vi "[FPGA] DeltaSig Main V6_5Mod.vi"() -> ()   [LabVIEW 2015]
doc: "This VI provides a template for customizing a waveform acquisition using delta-sigma based NI C Series analog input smodules."
uses:
  <vilib>/LabVIEW Targets/FPGA/cRIO/shared/nicrio_ModuleControls/nicrio_cRIO-9234_ConfigModeRing.ctl
  <vilib>/rvi/Emulation/niFpgaGetClockAttributes.vi
  <vilib>/rvi/Emulation/niFpgaSctlEmulationGetInTimedLoop.vi
  <vilib>/rvi/Emulation/niFpgaEmulationReportErrorSimple.vi
  <vilib>/LabVIEW Targets/FPGA/cRIO/shared/nicrio_DsaDataRateApi/_nicrio_9234GetDataRate131.vi
  <vilib>/rvi/Emulation/niFpgaProcessEmulError.vi
  <vilib>/rvi/eio/common/nirviEmuTemplatePropertySet_errors.vi
  <vilib>/rvi/eio/common/nirviEmuTemplateMethod_errors.vi
  <vilib>/rvi/interface/RandomDataEmulation/niFpgaRandomDataHandleErrors.vi
  <vilib>/rvi/Emulation/niFpgaCriticalErrorInLSC.vi
  <vilib>/eio/EIOPropertyNode/EIOPropertyNode.xnode
  <vilib>/LabVIEW Targets/FPGA/cRIO/shared/nicrio_ModuleControls/nicrio_cRIO-9234_DataRatesRing2.ctl
  <vilib>/eio/EIONode/EIONode.xnode
  <vilib>/rvi/DataTransferAndStorage/Container/XNode/niFpgaContainer.xnode
  <vilib>/rvi/interface/RandomDataEmulation/nirviRandomDataFpgaReadWriteTemplate.vi
  <vilib>/rvi/eio/common/nirviEmuTemplatePropertyGet_errors.vi
  <vilib>/rvi/eio/common/nirviEmuTemplatePropertyGet_noerrors.vi
  <vilib>/rvi/eio/common/nirviEmuTemplatePropertySet_noerrors.vi
panel:
  in  "Array Input Config":T1[](array[typedef])=[0, 0, 0, 0, 0, 0, 0, 0, 0, 0, 0, 0, 0, 0, 0, 0, 0, 0, 0, 0, 0, 0, 0, 0] items=["AC Coupled", "DC Coupled", "IEPE AC Coupled"]
  out "oclk freq":u32
  out "oclk div":u32
  out "oclk mult":u32
  in  "data rate (S/s)":u32
  in  "Chan Scale Array":sgl[](array[numeric])=[0.0, 0.0, 0.0, 0.0, 0.0, 0.0, 0.0, 0.0, 0.0, 0.0, 0.0, 0.0, 0.0, 0.0, 0.0, 0.0, 0.0, 0.0, 0.0, 0.0, 0.0, 0.0, 0.0, 0.0, 0.0, 0.0, 0.0, 0.0, 0.0, 0.0, 0.0, 0.0, 0.0, 0.0, 0.0, 0.0, 0.0, 0.0, 0.0, 0.0]
  out "Chan Count":bool
  out "Acq Loop Ticks":u32
  out "FPGA Error":errorcluster
  out "Module Underflow":bool
  out "Finished":bool
  in  "Number of Channels":i32=24
  in  "Samps per Chan [Finite]":i32=5120
  out "First Read":bool
  in  "Acquisition Type":enum16{"Finite Samples", "Continuous Samples"}(ring)
  out "DMA FIFO Full":bool
  in  "stop":bool
  # "Array size fixed at 40\nelements but may be \nexpanded if needed"
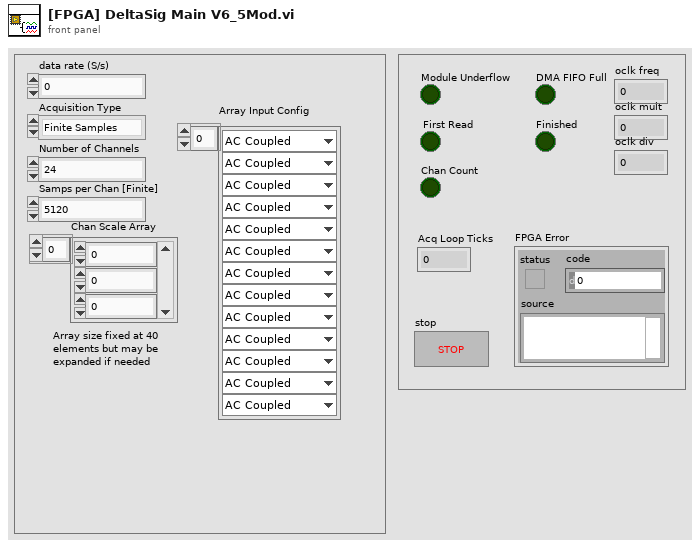
[diagram p1: front panel]
types:
  T1 = typedef "nicrio_cRIO-9234_ConfigModeRing.ctl" = u8
  T2 = typedef "nicrio_cRIO-9234_DataRatesRing2.ctl" = u8
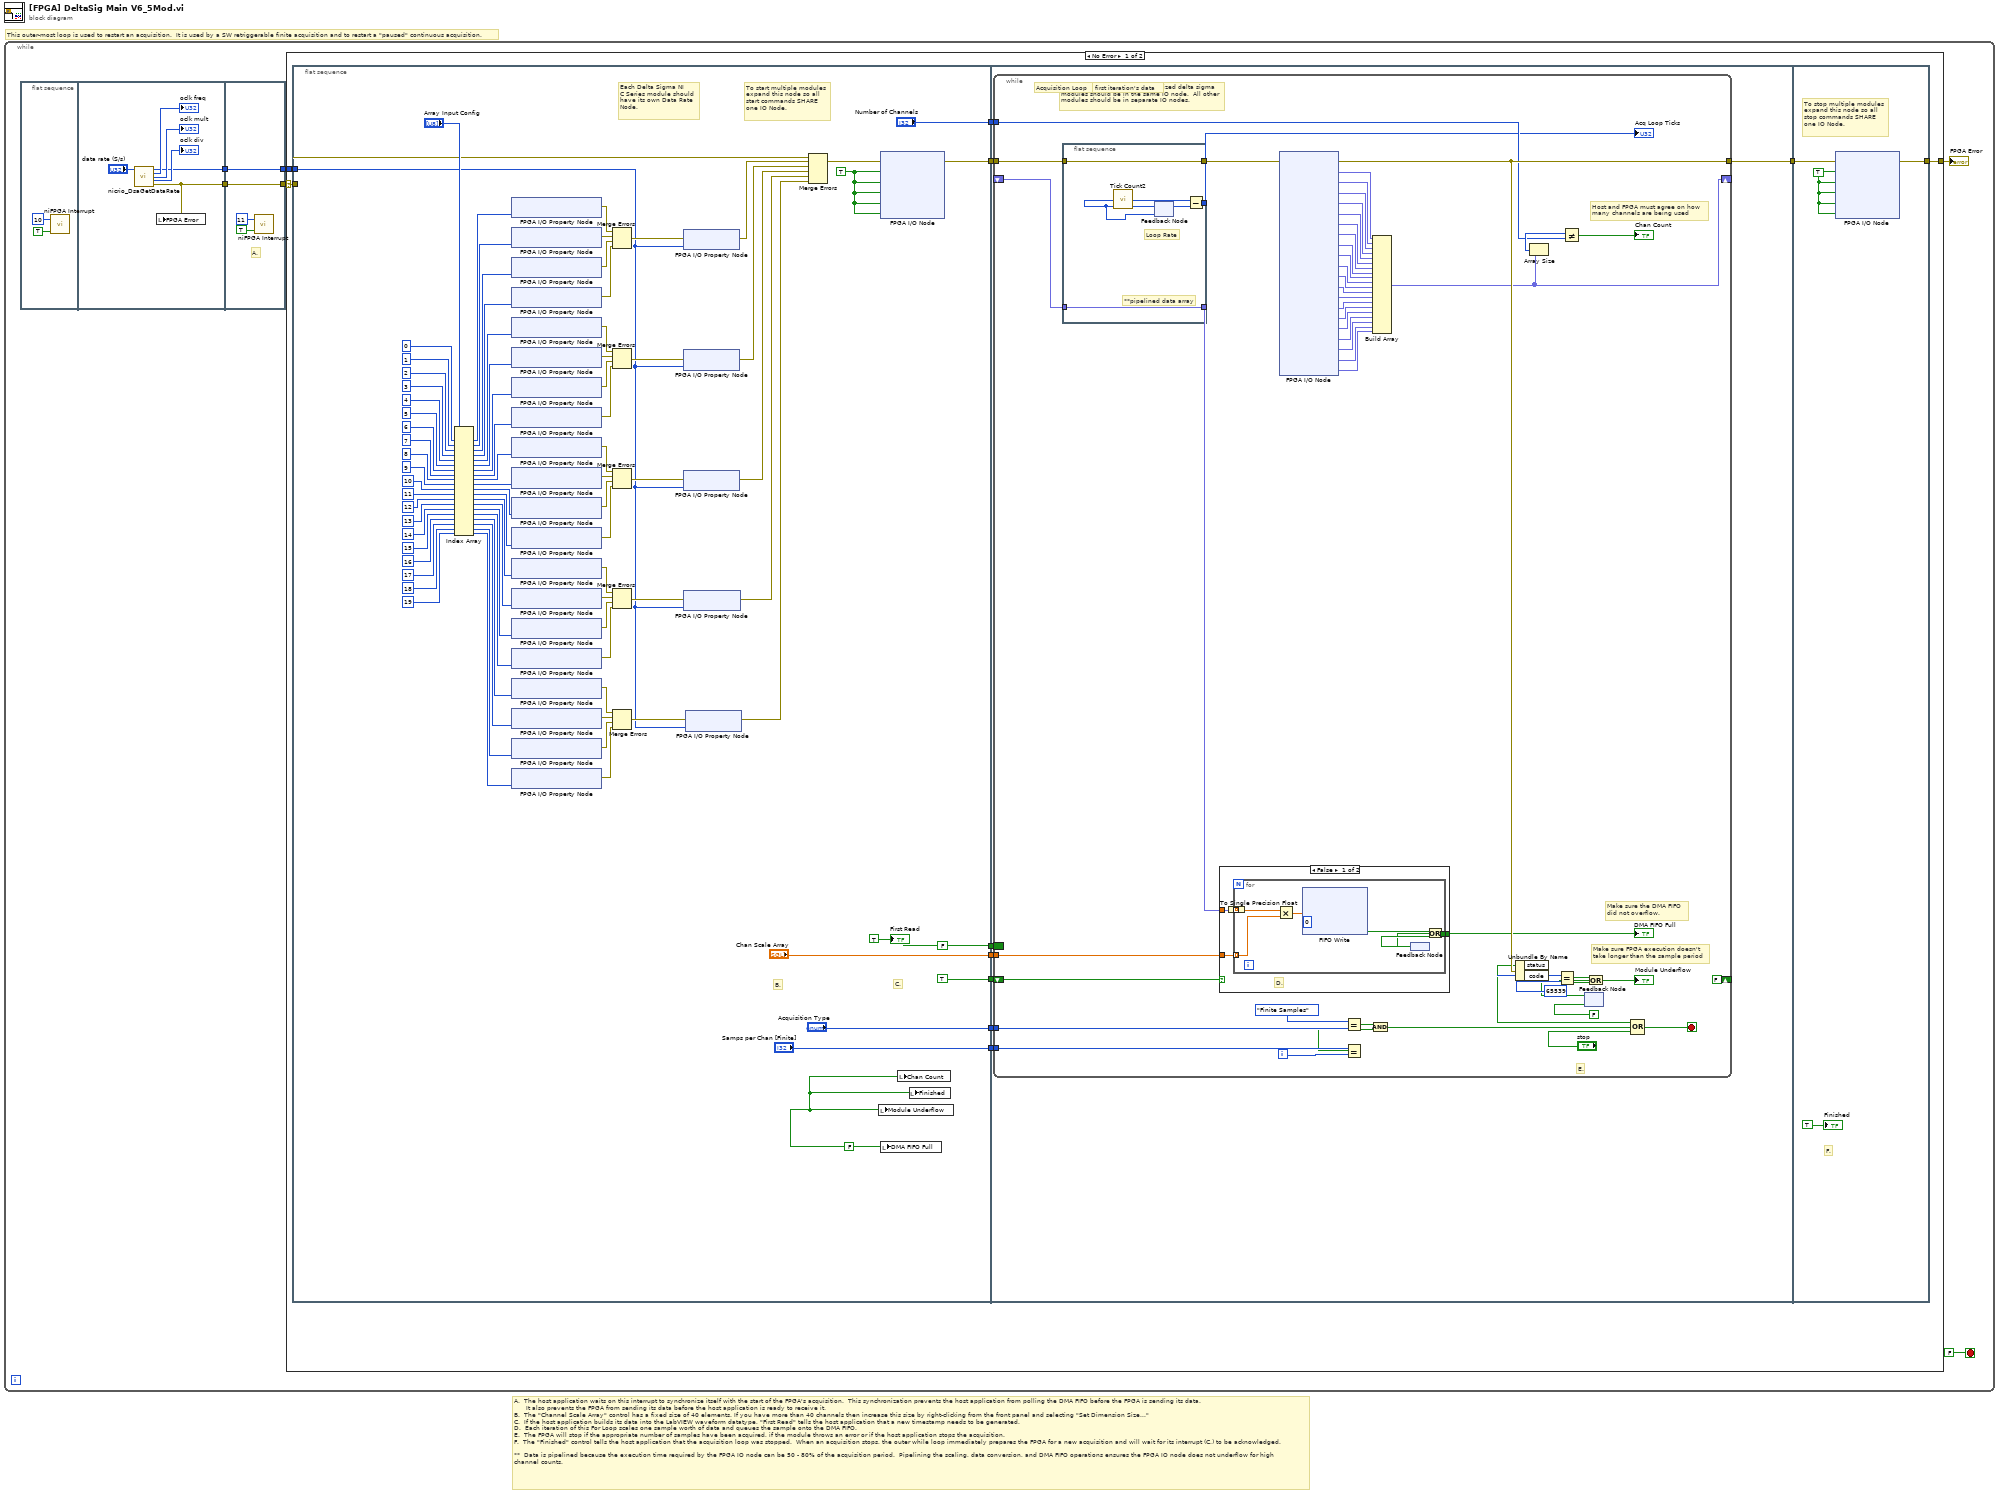
[diagram p0: block diagram]
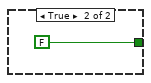
[diagram p2: hidden frame]
diagram:
  # "A.  The host application waits on this interrupt to synchronize itself with the start of the FPGA's acquisition.  This synchronization prevents the host application from polling the DMA FIFO before the FPGA is sending its data.\n      It also prevents the FPGA from sending its data before the host application is ready to receive it.\nB.  The \"Channel Scale Array\" control has a fixed size of 40 elements. If you have more than 40 channels then increase this size by right-clicking from the front panel and selecting \"Set Dimension Size...\"\nC.  If the host application builds its data into the LabVIEW waveform datatype, \"First Read\" tells the host application that a new timestamp needs to be generated.\nD.  Each iteration of this For Loop scales one sample worth of data and queues the sample onto the DMA FIFO.  \nE.  The FPGA will stop if the appropriate number of samples have been acquired, if the module throws an error or if the host application stops the acquisition.  \nF.  The \"Finished\" control tells the host application that the acquisition loop was stopped.  When an acquisition stops, the outer while loop immediately prepares the FPGA for a new acquisition and will wait for its interrupt (C.) to be acknowledged.\n\n**  Data is pipelined because the execution time required by the FPGA IO node can be 50 - 80% of the acquisition period.  Pipelining the scaling, data conversion, and DMA FIFO operations ensures the FPGA IO node does not underflow for high\nchannel counts."
  # "This outer-most loop is used to restart an acquisition.  It is used by a SW retriggerable finite acquisition and to restart a \"paused\" continuous acquisition."
  n1 = while {
    stop <- FALSE stop-if-true
    n2 = flat-sequence {
      tunnel: [w10] -> w2
      tunnel: [w11] -> w1
      tunnel: [w18] -> w3
      tunnel: [w15] -> w4
      tunnel: w2 -> [w15]
      tunnel: w1 -> [w18]
      frame #0 {
        n3 = call <vilib>:"niFPGA Interrupt.vi"("Wait Until Cleared (F)"=TRUE ("Wait Until Cleared"), "IRQ Number (0)"=u8 10 ("IRQ Number")) -> ()  [unwired: 1 in]
      }
      frame #1 {
        n4 = call-poly <vilib>:"nicrio_DsaGetDataRate.vi"("data rate (S/s)"="data rate (S/s)") -> ("data rate"=w11:T2, "oclk freq"=→"oclk freq":u32, "oclk mult"=→"oclk mult":u32, "oclk div"=→"oclk div":u32, "error out"=w10:errorcluster)  [unwired: 10 in]
        n5 = local write "FPGA Error"(w10) -> ()
      }
      frame #2 {
        # "A."
        n6 = call <vilib>:"niFPGA Interrupt.vi"("Wait Until Cleared (F)"=TRUE ("Wait Until Cleared"), "IRQ Number (0)"=u8 11 ("IRQ Number")) -> ()  [unwired: 1 in]
      }
    }
    n7 = case shown="No Error" w4 {
      selector: w4 -> [w19 w193]
      tunnel: [w21 w193] -> w5
      tunnel: w3 -> [w20 _]
      frame No Error {
        n8 = flat-sequence {
          tunnel: [w113] -> w29
          tunnel: ["Chan Scale Array"] -> w28
          tunnel: ["Acquisition Type"] -> w27
          tunnel: ["Samps per Chan [Finite]"] -> w26
          tunnel: ["Number of Channels"] -> w25
          tunnel: [TRUE ("t")] -> w24
          tunnel: [FALSE] -> w23
          tunnel: w20 -> [w33]
          tunnel: w19 -> [w85]
          tunnel: w29 -> [w120]
          tunnel: w28 -> [w119]
          tunnel: w27 -> [w117]
          tunnel: w26 -> [w116]
          tunnel: w25 -> [w121]
          tunnel: w24 -> [w118]
          tunnel: [w115] -> w22
          tunnel: w23 -> [w114]
          tunnel: w22 -> [w191]
          tunnel: [w190] -> w21
          frame #0 {
            w111 = FALSE ("Module Underflow")
            w73 = TRUE ("Mod1/Start")
            # "To start multiple modules\nexpand this node so all\nstart commands SHARE\none IO Node."
            # "C."
            # "B."
            # "Each Delta Sigma NI \nC Series module should \nhave its own Data Rate \nNode."
            n9 = Index Array(array="Array Input Config", index #1=0 ("index"), index #2=1 ("index"), index #3=2 ("index"), index #4=3 ("index"), index #5=4 ("index"), index #6=5 ("index"), index #7=6 ("index"), index #8=7 ("index"), index #9=8 ("index"), index #10=9 ("index"), index #11=10 ("index"), index #12=11 ("index"), index #13=12 ("index"), index #14=13 ("index"), index #15=14 ("index"), index #16=15 ("index"), index #17=16 ("index"), index #18=17 ("index"), index #19=18 ("index"), index #20=19 ("index")) -> (element #1=w103:T1, element #2=w102:T1, element #3=w101:T1, element #4=w100:T1, element #5=w81:T1, element #6=w80:T1, element #7=w79:T1, element #8=w78:T1, element #9=w60:T1, element #10=w59:T1, element #11=w58:T1, element #12=w57:T1, element #13=w56:T1, element #14=w54:T1, element #15=w53:T1, element #16=w52:T1, element #17=w51:T1, element #18=w50:T1, element #19=w49:T1, element #20=w48:T1)
            n10 = xnode "FPGA I/O Property Node"("Input Configuration"=w103) -> ("error out"=w96:errorcluster)  [unwired: 2 in, 1 out]
            n11 = xnode "FPGA I/O Property Node"("Input Configuration"=w102) -> ("error out"=w95:errorcluster)  [unwired: 2 in, 1 out]
            n12 = xnode "FPGA I/O Property Node"("Input Configuration"=w101) -> ("error out"=w94:errorcluster)  [unwired: 2 in, 1 out]
            n13 = xnode "FPGA I/O Property Node"("Input Configuration"=w100) -> ("error out"=w93:errorcluster)  [unwired: 2 in, 1 out]
            n14 = xnode "FPGA I/O Property Node"("Input Configuration"=w81) -> ("error out"=w90:errorcluster)  [unwired: 2 in, 1 out]
            n15 = xnode "FPGA I/O Property Node"("Input Configuration"=w80) -> ("error out"=w89:errorcluster)  [unwired: 2 in, 1 out]
            n16 = xnode "FPGA I/O Property Node"("Input Configuration"=w79) -> ("error out"=w88:errorcluster)  [unwired: 2 in, 1 out]
            n17 = xnode "FPGA I/O Property Node"("Input Configuration"=w78) -> ("error out"=w87:errorcluster)  [unwired: 2 in, 1 out]
            n18 = xnode "FPGA I/O Property Node"("Input Configuration"=w60) -> ("error out"=w72:errorcluster)  [unwired: 2 in, 1 out]
            n19 = xnode "FPGA I/O Property Node"("Input Configuration"=w59) -> ("error out"=w71:errorcluster)  [unwired: 2 in, 1 out]
            n20 = xnode "FPGA I/O Property Node"("Input Configuration"=w58) -> ("error out"=w70:errorcluster)  [unwired: 2 in, 1 out]
            n21 = xnode "FPGA I/O Property Node"("Input Configuration"=w57) -> ("error out"=w69:errorcluster)  [unwired: 2 in, 1 out]
            n22 = xnode "FPGA I/O Property Node"("Input Configuration"=w56) -> ("error out"=w68:errorcluster)  [unwired: 2 in, 1 out]
            n23 = xnode "FPGA I/O Property Node"("Input Configuration"=w54) -> ("error out"=w67:errorcluster)  [unwired: 2 in, 1 out]
            n24 = xnode "FPGA I/O Property Node"("Input Configuration"=w53) -> ("error out"=w66:errorcluster)  [unwired: 2 in, 1 out]
            n25 = xnode "FPGA I/O Property Node"("Input Configuration"=w52) -> ("error out"=w65:errorcluster)  [unwired: 2 in, 1 out]
            n26 = xnode "FPGA I/O Property Node"("Input Configuration"=w51) -> ("error out"=w64:errorcluster)  [unwired: 2 in, 1 out]
            n27 = xnode "FPGA I/O Property Node"("Input Configuration"=w50) -> ("error out"=w63:errorcluster)  [unwired: 2 in, 1 out]
            n28 = xnode "FPGA I/O Property Node"("Input Configuration"=w49) -> ("error out"=w62:errorcluster)  [unwired: 2 in, 1 out]
            n29 = xnode "FPGA I/O Property Node"("Input Configuration"=w48) -> ("error out"=w61:errorcluster)  [unwired: 2 in, 1 out]
            n30 = Merge Errors(w96, w95, w94, w93) -> (w92:errorcluster)
            n31 = Merge Errors(w90, w89, w88, w87) -> (w86:errorcluster)
            n32 = Merge Errors(w72, w71, w70, w69) -> (w55:errorcluster)
            n33 = Merge Errors(w68, w67, w66, w65) -> (w35:errorcluster)
            n34 = Merge Errors(w64, w63, w62, w61) -> (w34:errorcluster)
            n35 = xnode "FPGA I/O Property Node"("error in"=w92, "Data Rate"=w33) -> ("error out"=w83:errorcluster)  [unwired: 1 in, 1 out]
            n36 = xnode "FPGA I/O Property Node"("error in"=w86, "Data Rate"=w33) -> ("error out"=w82:errorcluster)  [unwired: 1 in, 1 out]
            n37 = xnode "FPGA I/O Property Node"("error in"=w55, "Data Rate"=w33) -> ("error out"=w32:errorcluster)  [unwired: 1 in, 1 out]
            n38 = xnode "FPGA I/O Property Node"("error in"=w35, "Data Rate"=w33) -> ("error out"=w31:errorcluster)  [unwired: 1 in, 1 out]
            n39 = xnode "FPGA I/O Property Node"("error in"=w34, "Data Rate"=w33) -> ("error out"=w30:errorcluster)  [unwired: 1 in, 1 out]
            n40 = Merge Errors(w85, w83, w82, w32, w31, w30) -> (w84:errorcluster)
            n41 = local write "Module Underflow"(w111) -> ()
            n42 = xnode "FPGA I/O Node"("error in"=w84, "Mod1/Start"=w73, "Mod2/Start"=w73, "Mod3/Start"=w73, "Mod4/Start"=w73, "Mod5/Start"=w73) -> ("error out"=w113:errorcluster)  [unwired: 5 in, 5 out]
            n43 = local write "DMA FIFO Full"(w111) -> ()
            n44 = local write "Chan Count"(w111) -> ()
            n45 = local write "Finished"(w111) -> ()
            "First Read" <- TRUE ("First Read")
          }
          frame #1 {
            n46 = while {
              tunnel: w120 -> [w161]
              tunnel: [w166] -> w115
              tunnel: w117 -> [w168]
              tunnel: w116 -> [w167]
              shift-right: [w141] -> _
              shift-left: _ -> [w154]
              tunnel: w121 -> [w163]
              tunnel: w119 -> [w155]
              shift-right: [FALSE ("t")] -> _
              shift-left: w118 -> [w153]
              border: w114 -> [_]
              i -> [w151]
              stop <- w138 stop-if-true
              # "Add channels here.  All synchronized delta sigma\nmodules should be in the same IO node.  All other\nmodules should be in separate IO nodes."
              # "Do not DMA first iteration's data"
              # "Acquisition Loop"
              # "E."
              # "Host and FPGA must agree on how \nmany channels are being used"
              # "Make sure the DMA FIFO\ndid not overflow."
              # "Make sure FPGA execution doesn't\ntake longer than the sample period"
              n47 = flat-sequence {
                tunnel: [w188] -> w160
                tunnel: w161 -> [w188]
                tunnel: [w185] -> w159
                tunnel: w154 -> [w184]
                tunnel: [w184] -> w140
                frame #0 {
                  # "**pipelined data array"
                  # "Loop Rate"
                  n48 = call "Tick Count2"() -> ("Tick Count(Ticks)"=w187:u32)
                  n49 = feedback-in #1(w187) -> ()
                  n50 = feedback #1(w187) -> (w186:u32)
                  n51 = Subtract(x=w187, y=w186) -> (x-y=w185:u32)
                }
              }
              n52 = To Single Precision Float(number=w140) -> (single precision float=w139:sgl[])
              n53 = case shown="False" w153 {
                tunnel: [w175 FALSE] -> w165
                tunnel: w155 -> [w174 _]
                tunnel: w139 -> [w173 _]
                frame False {
                  # "D."
                  n54 = for {
                    tunnel: [w180] -> w175
                    tunnel: w173 -> [w178] mode=indexing
                    tunnel: w174 -> [w177] mode=indexing
                    n55 = Multiply(x=w178, y=w177) -> (x*y=w176:sgl)
                    n56 = xnode ("FIFO Write")("Element"=w176, "Timeout"=0) -> ("Timed Out?"=w182:bool)  [unwired: 1 in, 1 out]
                    n57 = feedback #2() -> (w181:bool)
                    n58 = Or(x=w182, y=w181) -> (x .or. y?=w180:bool)
                    n59 = feedback-in #2(w180) -> ()
                  }
                }
                frame True {
                }
              }
              "DMA FIFO Full" <- w165
              n60 = xnode "FPGA I/O Node"("error in"=w160) -> ("error out"=w166:errorcluster, "Mod1/AI0"=w158:fxp<+/-,24,4>, "Mod1/AI1"=w150:fxp<+/-,24,4>, "Mod1/AI2"=w157:fxp<+/-,24,4>, "Mod1/AI3"=w156:fxp<+/-,24,4>, "Mod2/AI0"=w137:fxp<+/-,24,4>, "Mod2/AI1"=w136:fxp<+/-,24,4>, "Mod2/AI2"=w135:fxp<+/-,24,4>, "Mod2/AI3"=w134:fxp<+/-,24,4>, "Mod3/AI0"=w133:fxp<+/-,24,4>, "Mod3/AI1"=w132:fxp<+/-,24,4>, "Mod3/AI2"=w131:fxp<+/-,24,4>, "Mod3/AI3"=w130:fxp<+/-,24,4>, "Mod4/AI0"=w129:fxp<+/-,24,4>, "Mod4/AI1"=w128:fxp<+/-,24,4>, "Mod4/AI2"=w127:fxp<+/-,24,4>, "Mod4/AI3"=w126:fxp<+/-,24,4>, "Mod5/AI0"=w125:fxp<+/-,24,4>, "Mod5/AI1"=w124:fxp<+/-,24,4>, "Mod5/AI2"=w123:fxp<+/-,24,4>, "Mod5/AI3"=w122:fxp<+/-,24,4>)  [unwired: 20 in, 20 out]
              n61 = Equal?(x=enum16{"Finite Samples", "Continuous Samples"}."Finite Samples" ("y"), y=w168) -> (x = y?=w144:bool)
              n62 = Equal?(x=w167, y=w151) -> (x = y?=w143:bool)
              n63 = And(x=w144, y=w143) -> (x .and. y?=w142:bool)
              n64 = Build Array(w158, w150, w157, w156, w137, w136, w135, w134, w133, w132, w131, w130, w129, w128, w127, w126, w125, w124, w123, w122) -> (w141:fxp<+/-,24,4>[])
              n65 = Unbundle By Name(w166) -> ("status"=w149:bool, "code"=w169:i32)
              n66 = Array Size(array=w141) -> (size(s)=w164:i32)
              n67 = Equal?(x=w169, y=65539) -> (x = y?=w146:bool)
              n68 = Not Equal?(x=w164, y=w163) -> (x != y?=→"Chan Count":bool)
              n69 = feedback #3(FALSE) -> (w148:bool)
              n70 = Or(x=w146, y=w148) -> (x .or. y?=w145:bool)
              "Module Underflow" <- w145
              n71 = feedback-in #3(w145) -> ()
              n72 = Compound Arithmetic op=OR(w149, w142, "stop") -> (w138:bool)
              "Acq Loop Ticks" <- w159
            }
          }
          frame #2 {
            w189 = TRUE ("Mod1/Stop")
            # "To stop multiple modules\nexpand this node so all\nstop commands SHARE\none IO Node."
            # "F."
            n73 = xnode "FPGA I/O Node"("error in"=w191, "Mod1/Stop"=w189, "Mod2/Stop"=w189, "Mod3/Stop"=w189, "Mod4/Stop"=w189, "Mod5/Stop"=w189) -> ("error out"=w190:errorcluster)  [unwired: 5 in, 5 out]
            "Finished" <- TRUE ("Finished")
          }
        }
      }
      frame Error {
      }
    }
    "FPGA Error" <- w5
  }
